vi "ID FGV.vi"(11 "FGV State":T1) -> (3 "Value":i32)   [LabVIEW 2013, in "LVH-XBMC.lvlib"]
uses:
  LVH-XBMC.lvlib
  Type Defs/ID FGV State.ctl
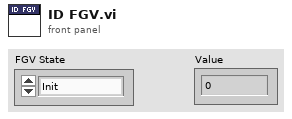
[diagram p1: front panel]
types:
  T1 = typedef "LVH-XBMC.lvlib/ID FGV State.ctl" = enum16{"Init", "Peek", "Get++"}
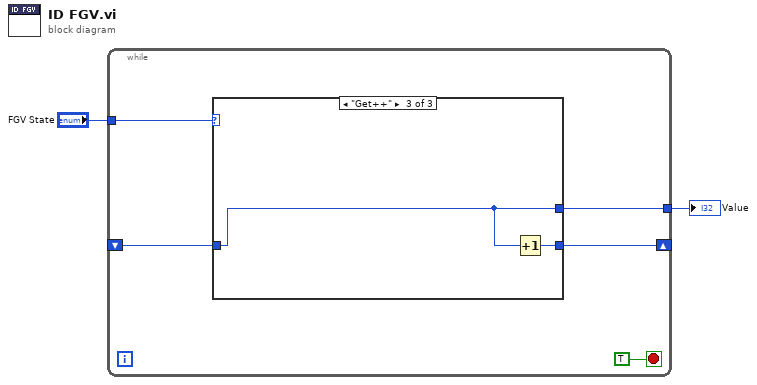
[diagram p0: block diagram]
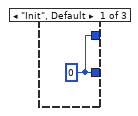
[diagram p2: hidden frame]
diagram:
  n1 = while {
    tunnel: "FGV State" -> [w6]
    shift-right: [w5] -> _
    shift-left: _ -> [w4]
    tunnel: [w3] -> w1
    stop <- TRUE stop-if-true
    n2 = case shown="\"Get++\"" w6 {
      tunnel: [w8 w9 w11] -> w5
      tunnel: w4 -> [_ w9 w10]
      tunnel: [w8 w9 w10] -> w3
      frame "Init", Default {
        w8 = 0 ("id")
      }
      frame "Peek" {
      }
      frame "Get++" {
        n3 = Increment(x=w10) -> (x+1=w11:i32)
      }
    }
  }
  "Value" <- w1
